vi "Build Scalar Channel Dictionary.vi"(8 "error in (no error)":errorcluster, 11 "scalar channels":T1[](array[typedef]) {"Data Type" format="%.0x"}) -> (0 "error out":errorcluster, 3 "scalar channels dictionary":variant)   [LabVIEW 2020, in "FPGA Addon System Explorer.lvlib"]
uses:
  FPGA Addon System Explorer.lvlib
  Addon Shared/Types/Register Information.ctl
  Addon Shared/Types/FPGA Addon Data Type.ctl
  Addon Shared/FPGA Addon Shared.lvlib
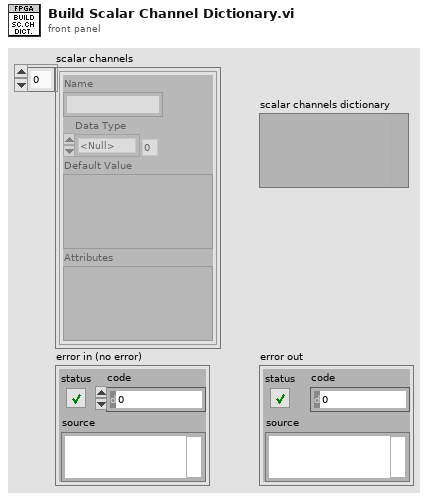
[diagram p1: front panel]
types:
  T1 = typedef "FPGA Addon Shared.lvlib/Register Information.ctl" = cluster{"Name":string, "Data Type":T2, "Default Value":variant, "Attributes":variant}
  T2 = typedef "FPGA Addon Shared.lvlib/FPGA Addon Data Type.ctl" = enum8{"<Null>", "I8", "I16", "I32", "I64", "U8", "U16", "U32", "U64", "SGL", "Boolean", "Analog PWM In Settings", "Analog PWM In", "Digital PWM In Settings", "Digital PWM In", "Digital PWM Out", "Sine Out", "FXP", "FXP+/-24.5", "FXP+/-16.5", "FXP+/-32.8", "FXP+/-64.32", "FXP+/-16.7", "FXP+/-20.5", "FXP+/-27.5", "FXP+/-32.16", "FXP+16.3", "FXP+18.3", "Digital Static In", "Digital Static Out", "Digital Static In Settings", "Digital WSS Out", "Quad Encoder Settings", "Quad Encoder In", "Group"}
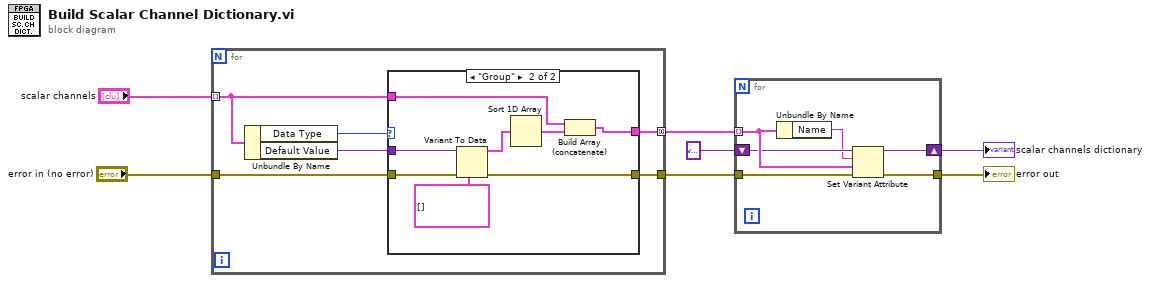
[diagram p0: block diagram]
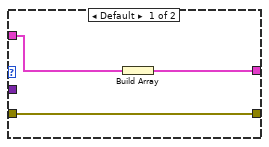
[diagram p2: hidden frame]
diagram:
  n1 = for {
    tunnel: "scalar channels" -> [w12] mode=indexing
    tunnel: "error in (no error)" -> [w9]
    tunnel: [w11] -> w3 mode=concatenating
    tunnel: [w8] -> w4
    n2 = Unbundle By Name(w12) -> ("Data Type"=w13:T2, "Default Value"=w10:variant)
    n3 = case shown="\"Group\"" w13 {
      tunnel: w12 -> [w16 w18]
      tunnel: [w15 w17] -> w11
      tunnel: w10 -> [_ w22]
      tunnel: w9 -> [w14 w21]
      tunnel: [w14 w20] -> w8
      frame Default {
        n4 = Build Array(w16) -> (w15:T1[])
      }
      frame "Group" {
        n5 = Variant To Data(error in=w21, type=T1[] [], Variant=w22) -> (data=w23:T1[], error out=w20:errorcluster)
        n6 = Sort 1D Array(array=w23) -> (sorted array=w19:T1[])
        n7 = Build Array (concatenate)(w18, w19) -> (w17:T1[])
      }
    }
  }
  n8 = for {
    tunnel: w3 -> [w30] mode=indexing
    tunnel: w4 -> [w29]
    tunnel: [w28] -> w5
    shift-right: [w27] -> w6
    shift-left: variant -> [w26]
    n9 = Unbundle By Name(w30) -> ("Name"=w25:string)
    n10 = Set Variant Attribute(Variant=w26, name=w25, value=w30, error in=w29) -> (Variant out=w27:variant, error out=w28:errorcluster)  [unwired: 1 out]
  }
  "error out" <- w5
  "scalar channels dictionary" <- w6
